vi "FPGA Target 2.vi"() -> ()   [LabVIEW 2025]
uses:
  <vilib>/Platform/TimedLoop/XDataNode/wakeup.ctl
  <vilib>/Platform/TimedLoop/XDataNode/XDNodeRunTimeDep.lvlib
  <vilib>/Platform/TimedLoop/XDataNode/nitl_modes.ctl
  <vilib>/Platform/TimedLoop/XDataNode/timing_clust.ctl
  <vilib>/Platform/TimedLoop/XDataNode/XDataNode.xnode
  SubModules/Engine Simulation Toolkit FPGA IP/IP Source/APU/APU.lvlib
  <vilib>/rvi/DataTransferAndStorage/Container/XNode/niFpgaContainer.xnode
  Templates/FPGA Wizard Templates.lvlib
  <vilib>/rvi/interface/RandomDataEmulation/nirviRandomDataFpgaReadWriteTemplate.vi
  SubModules/Engine Simulation Toolkit FPGA IP/IP Source/Digital Pattern Generation/Digital Pattern Generation.lvlib
  SubModules/Engine Simulation Toolkit FPGA IP/IP Source/Directional Speed/Directional Speed.lvlib
  SubModules/Engine Simulation Toolkit FPGA IP/IP Source/Analog Replay/Analog Replay.lvlib
  SubModules/FPGA Addon Speciality IO/Source/Speciality FPGA IO.lvlib
  SubModules/Engine Simulation Toolkit FPGA IP/IP Source/Knock Sensor/Knock Sensor.lvlib
  SubModules/Engine Simulation Toolkit FPGA IP/IP Source/ECU Event/Timing/ECU Event Timing.lvlib
  SubModules/Engine Simulation Toolkit FPGA IP/IP Source/ECU Event/Timing/Measure Events (Non-40MHz).vi
  SubModules/Engine Simulation Toolkit FPGA IP/IP Source/ECU Event/Timing/Capture Settings.ctl
  SubModules/Engine Simulation Toolkit FPGA IP/IP Source/APU/Shared Settings.ctl
  SubModules/Engine Simulation Toolkit FPGA IP/IP Source/Version Token.ctl
  SubModules/Engine Simulation Toolkit FPGA IP/IP Source/Engine Simulation Toolkit.lvlib
  SubModules/Engine Simulation Toolkit FPGA IP/IP Source/APU/Settings.ctl
  SubModules/Engine Simulation Toolkit FPGA IP/IP Source/APU/Input.ctl
  SubModules/Engine Simulation Toolkit FPGA IP/IP Source/APU/Output.ctl
  SubModules/Engine Simulation Toolkit FPGA IP/IP Source/Digital Pattern Generation/Load Input.ctl
  SubModules/Engine Simulation Toolkit FPGA IP/IP Source/Directional Speed/Load Input.ctl
  SubModules/Engine Simulation Toolkit FPGA IP/IP Source/Analog Replay/Load Input.ctl
  SubModules/FPGA Addon Speciality IO/Source/Types/PWM.Measure.Analog.Settings.ctl
  SubModules/FPGA Addon Speciality IO/Source/Types/PWM.Measure.Analog.Measurement.ctl
  SubModules/Engine Simulation Toolkit FPGA IP/IP Source/Knock Sensor/Cylinder Settings.ctl
  SubModules/Engine Simulation Toolkit FPGA IP/IP Source/Knock Sensor/Cylinder Input.ctl
  SubModules/Engine Simulation Toolkit FPGA IP/IP Source/Knock Sensor/Generate Settings.ctl
  SubModules/Engine Simulation Toolkit FPGA IP/IP Source/Knock Sensor/Generate Input.ctl
  SubModules/Engine Simulation Toolkit FPGA IP/IP Source/Analog Replay/Settings.ctl
  SubModules/Engine Simulation Toolkit FPGA IP/IP Source/Analog Replay/Input.ctl
  SubModules/FPGA Addon Speciality IO/Source/Types/Sine.Generate.Settings.ctl
  SubModules/FPGA Addon Speciality IO/Source/Types/PWM.Generate.Digital.Settings.ctl
  SubModules/Engine Simulation Toolkit FPGA IP/IP Source/Digital Pattern Generation/Settings.ctl
  SubModules/Engine Simulation Toolkit FPGA IP/IP Source/Digital Pattern Generation/Input.ctl
  SubModules/Engine Simulation Toolkit FPGA IP/IP Source/Directional Speed/Settings.ctl
  SubModules/Engine Simulation Toolkit FPGA IP/IP Source/Directional Speed/Input.ctl
  SubModules/FPGA Addon Speciality IO/Source/Types/WSS.Generate.Digital.Settings.ctl
  SubModules/FPGA Addon Speciality IO/Source/Types/Static.Generate.Digital.Settings.ctl
  SubModules/FPGA Addon Speciality IO/Source/Types/PWM.Measure.Digital.Settings.ctl
  SubModules/FPGA Addon Speciality IO/Source/Types/PWM.Measure.Digital.Measurement.ctl
  SubModules/Engine Simulation Toolkit FPGA IP/IP Source/ECU Event/Timing/Measure Settings.ctl
  SubModules/Engine Simulation Toolkit FPGA IP/IP Source/ECU Event/Timing/Measure Output.ctl
  SubModules/Engine Simulation Toolkit FPGA IP/IP Source/ECU Event/Timing/Capture Output.ctl
  SubModules/FPGA Addon Speciality IO/Source/Types/Static.Measure.Digital.Settings.ctl
  SubModules/FPGA Addon Speciality IO/Source/Types/Static.Measure.Digital.Measurement.ctl
panel:
  out "Ign Power Loopback.Measure":T1
  in  "Ign Power Loopback.Settings":T2={"ACTIVE EDGE"=TRUE}
  out "Accessory Loopback.Measure":T1
  in  "Accessory Loopback.Settings":T2={"ACTIVE EDGE"=TRUE}
  out "Front Driver WS Loopback.Measure":T1
  in  "Front Driver WS Loopback.Settings":T2={"ACTIVE EDGE"=TRUE}
  out "Mod4.Monitor":bool[](array[boolean])
  out "Crank Loopback.Measure":T1
  in  "Crank Loopback.Settings":T2={"ACTIVE EDGE"=TRUE}
  out "Crank_Temp Loopback.Measure":T1
  in  "Crank_Temp Loopback.Settings":T2={"ACTIVE EDGE"=TRUE}
  out "Switch Loopback":bool
  out "Key Loopback":bool
  out "capture.Exhaust CAM 1 Loopback.Event 4":T3
  out "capture.Exhaust CAM 1 Loopback.Event 3":T3
  out "capture.Exhaust CAM 1 Loopback.Event 2":T3
  out "capture.Exhaust CAM 1 Loopback.Event 1":T3
  out "status.Exhaust CAM 1 Loopback":T4
  in  "settings.Exhaust CAM 1 Loopback":T5
  out "capture.Intake CAM 1 Loopback.Event 4":T3
  out "capture.Intake CAM 1 Loopback.Event 3":T3
  out "capture.Intake CAM 1 Loopback.Event 2":T3
  out "capture.Intake CAM 1 Loopback.Event 1":T3
  out "status.Intake CAM 1 Loopback":T4
  in  "settings.Intake CAM 1 Loopback":T5
  out "PWM Out 2 Loopback.Measure":T6
  in  "PWM Out 2 Loopback.Settings":T7={"ACTIVE EDGE"=TRUE, "TIMEOUT"=40000000}
  out "PWM Out 1 Loopback.Measure":T6
  in  "PWM Out 1 Loopback.Settings":T7={"ACTIVE EDGE"=TRUE, "TIMEOUT"=40000000}
  out "Mod3.Monitor":bool[](array[boolean])
  out "Mod2.Monitor":bool[](array[boolean])
  in  "Ign Power.Settings":T8={"ACTIVE EDGE"=TRUE, "OUTPUT"=FALSE}
  in  "Accessory.Settings":T8={"ACTIVE EDGE"=TRUE, "OUTPUT"=FALSE}
  in  "Front Driver WS.Settings":T9={"ACTIVE EDGE"=TRUE, "ACTIVE TICKS"=0, "INACTIVE TICKS"=0, "DATA"=0, "SENSOR TYPE"=0}
  out "Mod1.Monitor":bool[](array[boolean])
  in  "input.Crank":T10
  in  "settings.Crank":T11
  in  "input.Crank_Temp":T12
  in  "settings.Crank_Temp":T13
  in  "Switch":bool
  in  "Key":bool
  in  "input.Exhaust CAM 1":T12
  in  "settings.Exhaust CAM 1":T13
  in  "input.Intake CAM 1":T12
  in  "settings.Intake CAM 1":T13
  in  "PWM Out 2.Settings":T14={"ACTIVE EDGE"=TRUE, "ACTIVE TICKS"=0, "INACTIVE TICKS"=0}
  in  "PWM Out 1.Settings":T14={"ACTIVE EDGE"=TRUE, "ACTIVE TICKS"=0, "INACTIVE TICKS"=0}
  out "Mod5.Monitor":fxp<+/-,32,8>[](array[numeric])
  in  "Simple Knock 2.Settings":T15={"AMP"=0.0, "OFFSET"=0.0, "PERIODS/TICKS"=2.4999957531690598e-05}
  in  "Simple Knock 1.Settings":T15={"AMP"=0.0, "OFFSET"=0.0, "PERIODS/TICKS"=2.4999957531690598e-05}
  in  "input.VR Sensor2":T16
  in  "settings.VR Sensor2":T17
  in  "input.VR Sensor1":T16
  in  "settings.VR Sensor1":T17
  in  "Power Supply Setpoint":fxp<+/-,32,8> format="%#_27g"
  in  "Dyno Setpoint":fxp<+/-,32,8> format="%#_27g"
  in  "input.Knock2":T18
  in  "settings.Knock2":T19
  in  "input.Knock2.Cylinder 6":T20={"probability compare"=65535, "high freq scaler"=0.0, "trigger position"=0}
  in  "settings.Knock2.Cylinder 6":T21
  in  "input.Knock2.Cylinder 5":T20={"probability compare"=65535, "high freq scaler"=0.0, "trigger position"=0}
  in  "settings.Knock2.Cylinder 5":T21
  in  "input.Knock2.Cylinder 4":T20={"probability compare"=65535, "high freq scaler"=0.0, "trigger position"=0}
  in  "settings.Knock2.Cylinder 4":T21
  in  "input.Knock2.Cylinder 3":T20={"probability compare"=65535, "high freq scaler"=0.0, "trigger position"=0}
  in  "settings.Knock2.Cylinder 3":T21
  in  "input.Knock2.Cylinder 2":T20={"probability compare"=65535, "high freq scaler"=0.0, "trigger position"=0}
  in  "settings.Knock2.Cylinder 2":T21
  in  "input.Knock2.Cylinder 1":T20={"probability compare"=65535, "high freq scaler"=0.0, "trigger position"=0}
  in  "settings.Knock2.Cylinder 1":T21
  in  "input.Knock1":T18
  in  "settings.Knock1":T19
  in  "input.Knock1.Cylinder 6":T20={"probability compare"=65535, "high freq scaler"=0.0, "trigger position"=0}
  in  "settings.Knock1.Cylinder 6":T21
  in  "input.Knock1.Cylinder 5":T20={"probability compare"=65535, "high freq scaler"=0.0, "trigger position"=0}
  in  "settings.Knock1.Cylinder 5":T21
  in  "input.Knock1.Cylinder 4":T20={"probability compare"=65535, "high freq scaler"=0.0, "trigger position"=0}
  in  "settings.Knock1.Cylinder 4":T21
  in  "input.Knock1.Cylinder 3":T20={"probability compare"=65535, "high freq scaler"=0.0, "trigger position"=0}
  in  "settings.Knock1.Cylinder 3":T21
  in  "input.Knock1.Cylinder 2":T20={"probability compare"=65535, "high freq scaler"=0.0, "trigger position"=0}
  in  "settings.Knock1.Cylinder 2":T21
  in  "input.Knock1.Cylinder 1":T20={"probability compare"=65535, "high freq scaler"=0.0, "trigger position"=0}
  in  "settings.Knock1.Cylinder 1":T21
  out "Simple Knock 2 Loopback":fxp<+/-,32,8> format="%#_27g"
  out "Simple Knock 1 Loopback":fxp<+/-,32,8> format="%#_27g"
  out "VR Sensor2 Loopback.Measure":T22
  in  "VR Sensor2 Loopback.Settings":T23={"ACTIVE EDGE"=TRUE, "TIMEOUT"=40000000, "THRESHOLD"=50.0}
  out "VR Sensor1 Loopback.Measure":T22
  in  "VR Sensor1 Loopback.Settings":T23={"ACTIVE EDGE"=TRUE, "TIMEOUT"=40000000, "THRESHOLD"=50.0}
  out "Power Supply Setpoint Loopback":fxp<+/-,32,8> format="%#_27g"
  out "Dyno Setpoint Loopback":fxp<+/-,32,8> format="%#_27g"
  out "Knock2 Loopback":fxp<+/-,32,8> format="%#_27g"
  out "Knock1 Loopback":fxp<+/-,32,8> format="%#_27g"
  out "Mod6.Monitor":fxp<+/-,24,5>[](array[numeric])
  in  "load input.VR Sensor2":T24={"Data"=[0, 0, 0, 0, 0, 0, 0, 0, 0, 0, 0, 0, 0, 0, 0, 0], "LoadOffset"=0, "Done"=FALSE}
  in  "load input.VR Sensor1":T24={"Data"=[0, 0, 0, 0, 0, 0, 0, 0, 0, 0, 0, 0, 0, 0, 0, 0], "LoadOffset"=0, "Done"=FALSE}
  in  "load input.Crank":T25
  in  "load input.Crank_Temp":T26
  in  "load input.Exhaust CAM 1":T26
  in  "load input.Intake CAM 1":T26
  out "Actual Analog Input Loop Period (usec)":u32
  out "Actual Analog Output Loop Period (usec)":u32
  out "Actual Digital Loop Period (usec)":u32
  out "Actual DMA Loop Period (usec)":u32
  in  "Analog Input Loop Timer (uSec)":u32=10
  out "output.apu 1":T27 caption="output"
  in  "input.apu 1":T28={"desired speed"=0.0, "reset"=TRUE} caption="input"
  in  "settings.apu 1":T29 caption="settings"
  in  "est.version":T30
  in  "shared settings.apu 1":T31 {"start" format="%#.15g"}
  in  "go.apu 1":bool
  in  "Digital Loop Timer (uSec)":u32=10
  in  "Analog Output Loop Timer (uSec)":u32=10
  in  "DMA.Enable":bool
  in  "DMA.MinimumSamples":u32=100000 caption="DMA Loop Timer (uSec)"
  out "DMA.Timeout":bool
  in  "DMA.Timeout.Reset":bool
  in  "DMA Loop Timer (uSec)":u32=10
types:
  T1 = typedef "Speciality FPGA IO.lvlib/Static.Measure.Digital.Measurement.ctl" = cluster{"STATE":bool}
  T2 = typedef "Speciality FPGA IO.lvlib/Static.Measure.Digital.Settings.ctl" = cluster{"ACTIVE EDGE":bool}
  T3 = typedef "Engine Simulation Toolkit.lvlib/ECU Event Timing.lvlib/Capture Output.ctl" = cluster{"Start":u16, "End":u16, "Duration (tics)":fxp<+,18,18>, "Event present":bool}
  T4 = typedef "Engine Simulation Toolkit.lvlib/ECU Event Timing.lvlib/Measure Output.ctl" = cluster{"stuck active":bool, "window all active":bool, "window orphan start":bool, "window orphan end":bool}
  T5 = typedef "Engine Simulation Toolkit.lvlib/ECU Event Timing.lvlib/Measure Settings.ctl" = cluster{"max":u16, "min":u16, "active high":bool, "wrap":bool}
  T6 = typedef "Speciality FPGA IO.lvlib/PWM.Measure.Digital.Measurement.ctl" = cluster{"ACTIVE TICKS":u32, "INACTIVE TICKS":u32, "ACQ TICKS":u32}
  T7 = typedef "Speciality FPGA IO.lvlib/PWM.Measure.Digital.Settings.ctl" = cluster{"ACTIVE EDGE":bool, "TIMEOUT":u32}
  T8 = typedef "Speciality FPGA IO.lvlib/Static.Generate.Digital.Settings.ctl" = cluster{"ACTIVE EDGE":bool, "OUTPUT":bool}
  T9 = typedef "Speciality FPGA IO.lvlib/WSS.Generate.Digital.Settings.ctl" = cluster{"ACTIVE EDGE":bool, "ACTIVE TICKS":u32, "INACTIVE TICKS":u32, "DATA":u8, "SENSOR TYPE":u8}
  T10 = typedef "Engine Simulation Toolkit.lvlib/Directional Speed.lvlib/Input.ctl" = cluster{"td (tics)":u16, "tf (tics)":u16, "tr (tics)":u16}
  T11 = typedef "Engine Simulation Toolkit.lvlib/Directional Speed.lvlib/Settings.ctl" = cluster{"Upper Value":u16, "Lower Value":u16, "Upper Index":fxp<+,10,10>, "Lower Index":fxp<+,10,10>, "Enabled":bool}
  T12 = typedef "Engine Simulation Toolkit.lvlib/Digital Pattern Generation.lvlib/Input.ctl" = cluster{"Offset":i16}
  T13 = typedef "Engine Simulation Toolkit.lvlib/Digital Pattern Generation.lvlib/Settings.ctl" = cluster{"edge 1":u16, "edge 2":u16, "cycle angle":bool, "enabled":bool, "first falling":bool, "fault":bool, "fault wrap":bool, "fault value":bool, "fault count":fxp<+,4,4>, "use fault count":bool}
  T14 = typedef "Speciality FPGA IO.lvlib/PWM.Generate.Digital.Settings.ctl" = cluster{"ACTIVE EDGE":bool, "ACTIVE TICKS":u32, "INACTIVE TICKS":u32}
  T15 = typedef "Speciality FPGA IO.lvlib/Sine.Generate.Settings.ctl" = cluster{"AMP":fxp<+/-,32,8>, "OFFSET":fxp<+/-,32,8>, "PERIODS/TICKS":fxp<+,32,0>}
  T16 = typedef "Engine Simulation Toolkit.lvlib/Analog Replay.lvlib/Input.ctl" = cluster{"Offset":i16, "VScaleSlope":fxp<+,18,6>, "VScaleIntercept":fxp<+/-,18,3>}
  T17 = typedef "Engine Simulation Toolkit.lvlib/Analog Replay.lvlib/Settings.ctl" = cluster{"ReverseNegate":bool, "CycleAngle":bool, "SpeedThreshold":fxp<+/-,23,2>, "AOBelowThreshold":i16}
  T18 = typedef "Engine Simulation Toolkit.lvlib/Knock Sensor.lvlib/Generate Input.ctl" = cluster{"low freq scaler":fxp<+,10,0>}
  T19 = typedef "Engine Simulation Toolkit.lvlib/Knock Sensor.lvlib/Generate Settings.ctl" = cluster{"low freq (periods/tick)":fxp<+,32,0>, "high freq (periods/tick)":fxp<+,32,0>, "duration (1.25MHz tics)":fxp<+,18,18>, "low freq speed slope":fxp<+,16,-3>, "low freq speed intercept":fxp<+,10,-10>, "low freq by speed":bool}
  T20 = typedef "Engine Simulation Toolkit.lvlib/Knock Sensor.lvlib/Cylinder Input.ctl" = cluster{"probability compare":u16, "high freq scaler":fxp<+,10,0>, "trigger position":u16}
  T21 = typedef "Engine Simulation Toolkit.lvlib/Knock Sensor.lvlib/Cylinder Settings.ctl" = cluster{"seed":u16, "reset":bool}
  T22 = typedef "Speciality FPGA IO.lvlib/PWM.Measure.Analog.Measurement.ctl" = cluster{"ACTIVE TICKS":u32, "INACTIVE TICKS":u32, "ACQ TICKS":u32, "ACTIVE VOLTAGE":fxp<+/-,32,8>, "INACTIVE VOLTAGE":fxp<+/-,32,8>}
  T23 = typedef "Speciality FPGA IO.lvlib/PWM.Measure.Analog.Settings.ctl" = cluster{"ACTIVE EDGE":bool, "TIMEOUT":u32, "THRESHOLD":fxp<+/-,32,8>}
  T24 = typedef "Engine Simulation Toolkit.lvlib/Analog Replay.lvlib/Load Input.ctl" = cluster{"Data":i16[], "LoadOffset":u16, "Done":bool}
  T25 = typedef "Engine Simulation Toolkit.lvlib/Directional Speed.lvlib/Load Input.ctl" = cluster{"address":fxp<+,10,10>, "done":bool, "angle":u16}
  T26 = typedef "Engine Simulation Toolkit.lvlib/Digital Pattern Generation.lvlib/Load Input.ctl" = cluster{"address":fxp<+,11,11>, "done":bool, "angle":u16}
  T27 = typedef "Engine Simulation Toolkit.lvlib/APU.lvlib/Output.ctl" = cluster{"crank":u16, "cycle":u16, "actual speed":fxp<+/-,23,2>}
  T28 = typedef "Engine Simulation Toolkit.lvlib/APU.lvlib/Input.ctl" = cluster{"desired speed":fxp<+/-,23,2>, "reset":bool}
  T29 = typedef "Engine Simulation Toolkit.lvlib/APU.lvlib/Settings.ctl" = cluster{"acceleration":fxp<+,18,-20>, "enable accel":bool}
  T30 = typedef "Engine Simulation Toolkit.lvlib/Version Token.ctl" = cluster{"1.4.0":bool}
  T31 = typedef "Engine Simulation Toolkit.lvlib/APU.lvlib/Shared Settings.ctl" = cluster{"start":fxp<+,17,17>, "stuck limit":fxp<+,18,18>}
  T32 = typedef "XDNodeRunTimeDep.lvlib/timing_clust.ctl" = cluster{"Expected End [f-1]":u64, "Actual End [f-1]":u64, "Finished Late? [f-1]":bool, "Expected End [i-1]":u64, "Actual End [i-1]":u64, "Finished Late? [i-1]":bool, "Expected Start [i]":u64, "Actual Start [i]":u64, "Expected Start [f]":u64, "Actual Start [f]":u64, "Source Name":string, "Structure Name":string, "Period":i64, "Deadline":i64, "Offset":i64, "Start":i64, "Priority":i32, "Timeout":i32, "Mode":T33, "Wakeup Reason":T34, "Error":errorcluster, "Source Type":string, "Secondary Source Type":string, "Global End Time":u64, "Global Start Time":u64, "Frame Duration":u64, "Iteration Duration":u64, "Assigned CPU":i32, "I/O Scan Engine Mode":u32}
  T33 = typedef "XDNodeRunTimeDep.lvlib/nitl_modes.ctl" = enum32{"No Change", "Process missed periods, maintain original phase", "Discard missed periods, maintain original phase", "Process missed periods, ignore original phase", "Discard missed periods, ignore original phase"}
  T34 = typedef "XDNodeRunTimeDep.lvlib/wakeup.ctl" = enum32{"Normal", "Aborted", "Asynchronous wakeup", "Timing source error", "Timed loop error", "Timeout"}
  T35 = cluster{"DI 0":refnum<k21>, "DI 1":refnum<k21>, "DI 2":refnum<k21>, "DI 3":refnum<k21>, "DI 4":refnum<k21>, "DI 5":refnum<k21>, "DI 6":refnum<k21>, "DI 7":refnum<k21>}
  T36 = typedef "Engine Simulation Toolkit.lvlib/ECU Event Timing.lvlib/Capture Settings.ctl" = u8
  T37 = cluster{"DO 0":refnum<k21>, "DO 1":refnum<k21>, "DO 2":refnum<k21>, "DO 3":refnum<k21>, "DO 4":refnum<k21>, "DO 5":refnum<k21>, "DO 6":refnum<k21>, "DO 7":refnum<k21>}
  T38 = cluster{"AO 0":refnum<k21>, "AO 1":refnum<k21>, "AO 2":refnum<k21>, "AO 3":refnum<k21>, "AO 4":refnum<k21>, "AO 5":refnum<k21>, "AO 6":refnum<k21>, "AO 7":refnum<k21>, "AO 8":refnum<k21>, "AO 9":refnum<k21>, "AO 10":refnum<k21>, "AO 11":refnum<k21>, "AO 12":refnum<k21>, "AO 13":refnum<k21>, "AO 14":refnum<k21>, "AO 15":refnum<k21>}
  T39 = cluster{"AI 0":refnum<k21>, "AI 1":refnum<k21>, "AI 2":refnum<k21>, "AI 3":refnum<k21>, "AI 4":refnum<k21>, "AI 5":refnum<k21>, "AI 6":refnum<k21>, "AI 7":refnum<k21>, "AI 8":refnum<k21>, "AI 9":refnum<k21>, "AI 10":refnum<k21>, "AI 11":refnum<k21>, "AI 12":refnum<k21>, "AI 13":refnum<k21>, "AI 14":refnum<k21>, "AI 15":refnum<k21>}
  T40 = typedef "Engine Simulation Toolkit.lvlib/Digital Pattern Generation.lvlib/Load Data.ctl" = cluster{"max address":fxp<+,11,11>, "memory":refnum<k21>}
  T41 = typedef "Engine Simulation Toolkit.lvlib/Directional Speed.lvlib/Load Data.ctl" = cluster{"max address":fxp<+,10,10>, "Memory":refnum<k21>}
  T42 = typedef "Engine Simulation Toolkit.lvlib/APU.lvlib/Register Bus.ctl" = cluster{"Speed":refnum<k21>, "Crank Angle":refnum<k21>, "Cycle Angle":refnum<k21>, "Crank Count":refnum<k21>, "Cycle Count":refnum<k21>, "1.25 MHz Counter":refnum<k21>, "Crank Rollover":refnum<k21>, "Cycle Rollover":refnum<k21>, "shared settings":T31}
  T43 = typedef "Engine Simulation Toolkit.lvlib/Knock Sensor.lvlib/Triggered Cylinder Data.ctl" = cluster{"trigger knock":bool, "high freq scaler":fxp<+,10,0>}
  T44 = typedef "Engine Simulation Toolkit.lvlib/ECU Event Timing.lvlib/Measured Data.ctl" = cluster{"start":u16, "end":u16, "duration (tics)":fxp<+,18,18>, "window end":bool, "window begin":bool, "pulse end":bool, "pulse #":u8}
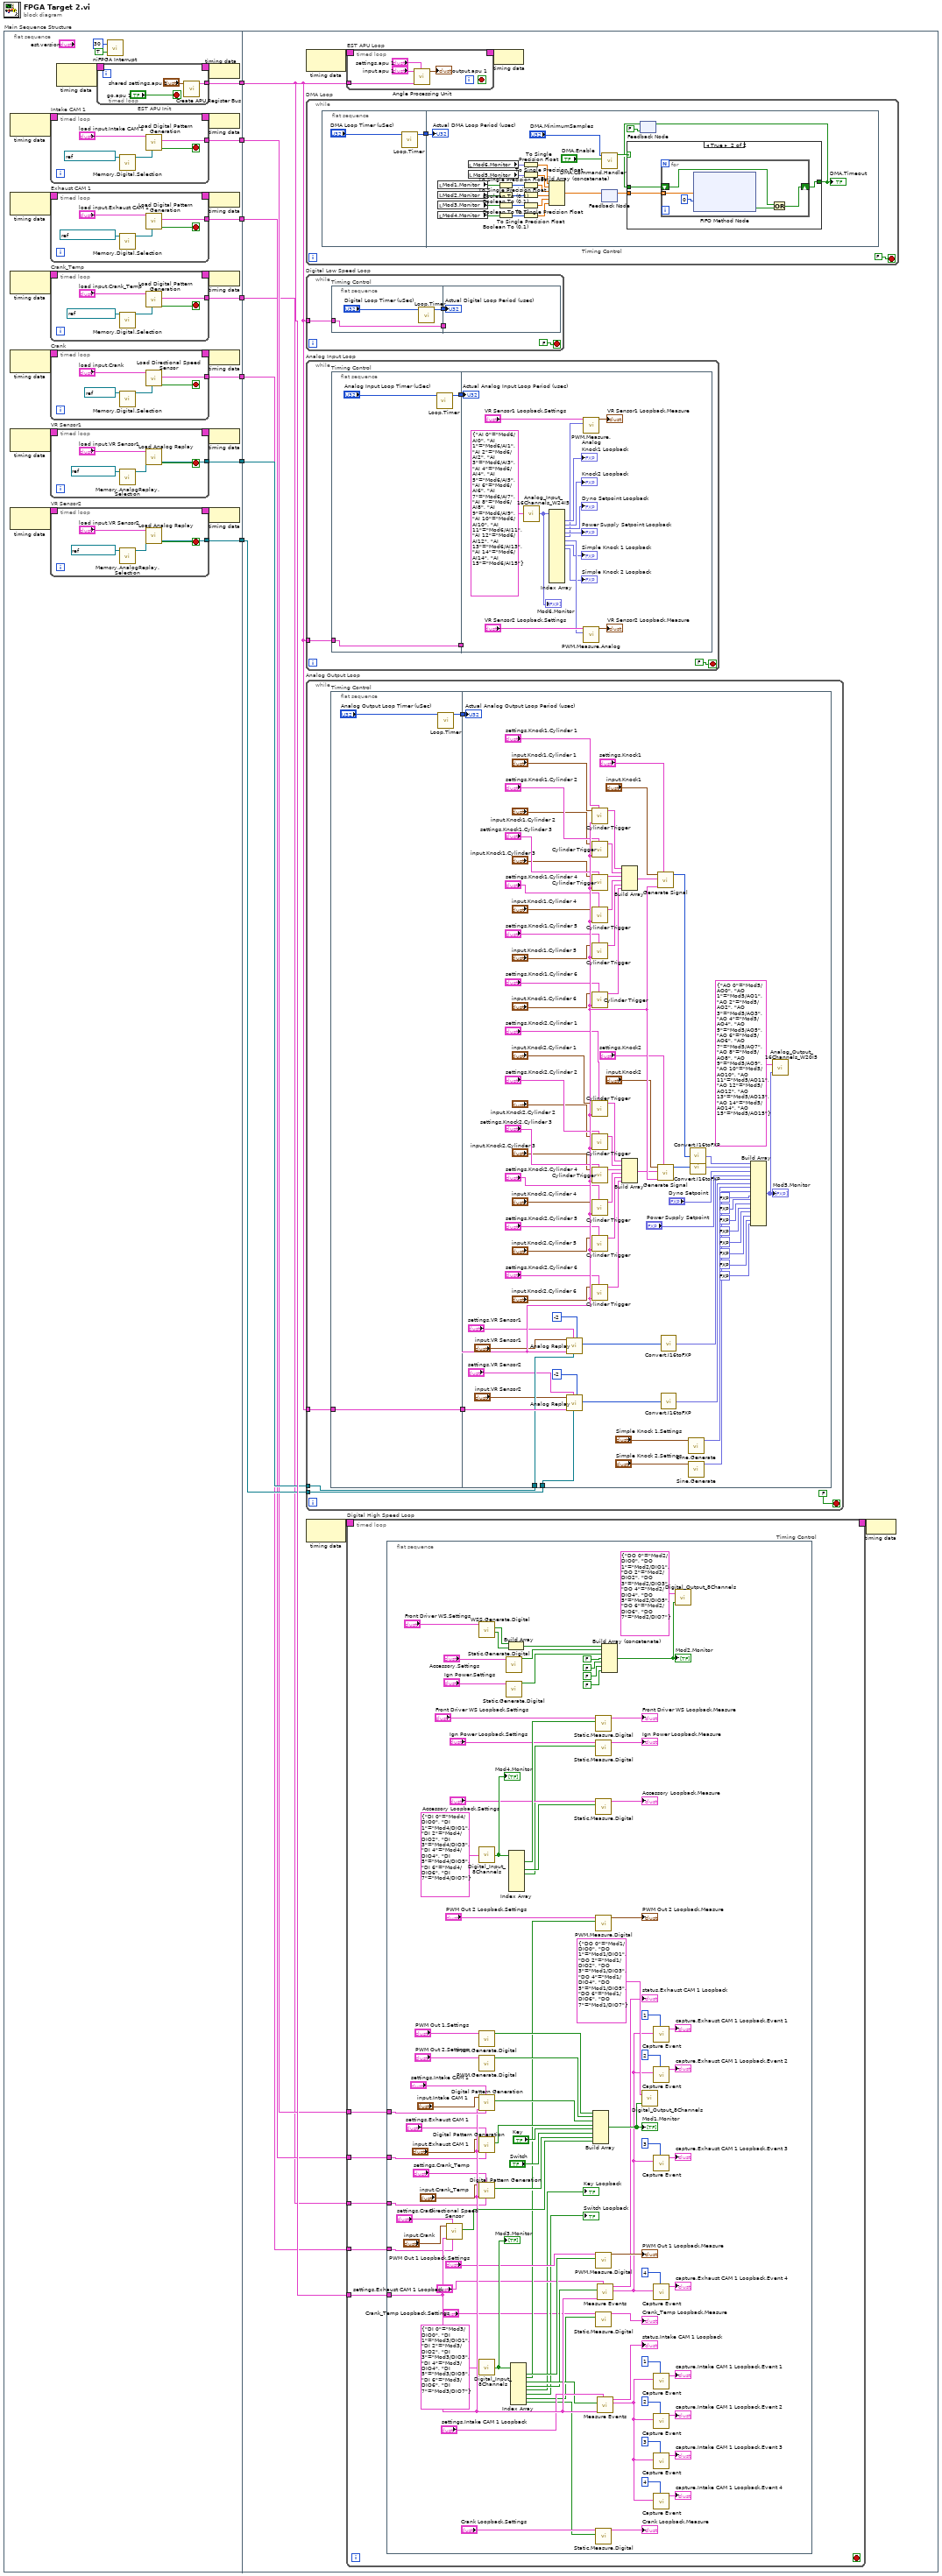
[diagram p0: block diagram]
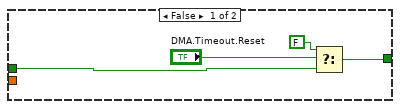
[diagram p2: hidden frame]
diagram:
  n1 = flat-sequence "Main Sequence Structure" {
    tunnel: [w26] -> w7
    tunnel: [w13] -> w6
    tunnel: [w12] -> w5
    tunnel: [w11] -> w4
    tunnel: [w10] -> w3
    tunnel: [w9] -> w2
    tunnel: [w8] -> w1
    tunnel: w7 -> [w96]
    tunnel: w6 -> [w95]
    tunnel: w5 -> [w94]
    tunnel: w4 -> [w93]
    tunnel: w3 -> [w92]
    tunnel: w2 -> [w91]
    tunnel: w1 -> [w90]
    frame #0 {
      n2 = node-c288() -> (w25:T32)  [unwired: 1 in]
      n3 = node-c288() -> (w23:T32)  [unwired: 1 in]
      n4 = node-c288() -> (w21:T32)  [unwired: 1 in]
      n5 = node-c288() -> (w19:T32)  [unwired: 1 in]
      n6 = node-c288() -> (w17:T32)  [unwired: 1 in]
      n7 = node-c288() -> (w15:T32)  [unwired: 1 in]
      n8 = timed-loop "Intake CAM 1" {
        timing: w25 -> [_]
        timing-out: [_] -> w24
        tunnel: [w74] -> w11
        stop <- w77 stop-if-true
        n9 = call "Memory.Digital.Selection.vi"("memory"=refnum<k21> "Intake CAM 1") -> ("memory"=w75:refnum<k21>)  [unwired: 10 in]
        n10 = call "Load Digital Pattern Generation.vi"("memory"=w75, "load input.<user name>"="load input.Intake CAM 1") -> ("done"=w77:bool, "load data"=w74:T40)  [unwired: 8 in]
      }
      n11 = timed-loop "Exhaust CAM 1" {
        timing: w23 -> [_]
        timing-out: [_] -> w22
        tunnel: [w65] -> w10
        stop <- w68 stop-if-true
        n12 = call "Memory.Digital.Selection.vi"("memory"=refnum<k21> "Exhaust CAM 1") -> ("memory"=w66:refnum<k21>)  [unwired: 10 in]
        n13 = call "Load Digital Pattern Generation.vi"("memory"=w66, "load input.<user name>"="load input.Exhaust CAM 1") -> ("done"=w68:bool, "load data"=w65:T40)  [unwired: 8 in]
      }
      n14 = timed-loop "Crank_Temp" {
        timing: w21 -> [_]
        timing-out: [_] -> w20
        tunnel: [w56] -> w9
        stop <- w59 stop-if-true
        n15 = call "Memory.Digital.Selection.vi"("memory"=refnum<k21> "Crank_Temp") -> ("memory"=w57:refnum<k21>)  [unwired: 10 in]
        n16 = call "Load Digital Pattern Generation.vi"("memory"=w57, "load input.<user name>"="load input.Crank_Temp") -> ("done"=w59:bool, "load data"=w56:T40)  [unwired: 8 in]
      }
      n17 = timed-loop "Crank" {
        timing: w19 -> [_]
        timing-out: [_] -> w18
        tunnel: [w47] -> w8
        stop <- w50 stop-if-true
        n18 = call "Memory.Digital.Selection.vi"("memory"=refnum<k21> "Crank") -> ("memory"=w48:refnum<k21>)  [unwired: 10 in]
        n19 = call "Load Directional Speed Sensor.vi"("Memory In"=w48, "load input.<user name>"="load input.Crank") -> ("done"=w50:bool, "load data"=w47:T41)  [unwired: 8 in]
      }
      n20 = timed-loop "VR Sensor1" {
        timing: w17 -> [_]
        timing-out: [_] -> w16
        tunnel: [w39] -> w13
        stop <- w41 stop-if-true
        n21 = call "Memory.AnalogReplay.Selection.vi"("memory"=refnum<k21> "VR Sensor1") -> ("memory"=w39:refnum<k21>)  [unwired: 10 in]
        n22 = call "Load Analog Replay.vi"("memory"=w39, "load input.<user name>"="load input.VR Sensor1") -> ("done"=w41:bool)  [unwired: 9 in]
      }
      n23 = timed-loop "VR Sensor2" {
        timing: w15 -> [_]
        timing-out: [_] -> w14
        tunnel: [w31] -> w12
        stop <- w33 stop-if-true
        n24 = call "Memory.AnalogReplay.Selection.vi"("memory"=refnum<k21> "VR Sensor2") -> ("memory"=w31:refnum<k21>)  [unwired: 10 in]
        n25 = call "Load Analog Replay.vi"("memory"=w31, "load input.<user name>"="load input.VR Sensor2") -> ("done"=w33:bool)  [unwired: 9 in]
      }
      n26 = node-c288() -> (w28:T32)  [unwired: 1 in]
      n27 = timed-loop "EST APU Init" {
        timing: w28 -> [_]
        timing-out: [_] -> w27
        tunnel: [w83] -> w26
        stop <- "go.apu 1" stop-if-true
        n28 = call "Create APU Register Bus.vi"("shared settings.<user name>"="shared settings.apu 1") -> ("register bus"=w83:T42)  [unwired: 10 in]
      }
      n29 = call <vilib>:"niFPGA Interrupt.vi"("Wait Until Cleared (F)"=TRUE, "IRQ Number (0)"=u8 30) -> ()  [unwired: 1 in]
      n30 = node-c288(w27) -> ()
      n31 = node-c288(w24) -> ()
      n32 = node-c288(w22) -> ()
      n33 = node-c288(w20) -> ()
      n34 = node-c288(w18) -> ()
      n35 = node-c288(w16) -> ()
      n36 = node-c288(w14) -> ()
    }
    frame #1 {
      # "FPGA Addon Code"
      n37 = node-c288 ("Input Node")() -> (w98:T32)  [unwired: 1 in]
      n38 = while "DMA Loop" {
        stop <- FALSE stop-if-true
        n39 = flat-sequence "Timing Control" {
          tunnel: [w210] -> w208
          tunnel: w208 -> [w228]
          frame #0 {
            n40 = call "Loop.Timer.vi"("Loop Timer (uSec)"="DMA Loop Timer (uSec)") -> ("Actual Loop Period (usec)"=w210:u32)  [unwired: 10 in]
          }
          frame #1 {
            n41 = local read "Mod1.Monitor"() -> (w225:bool[])
            n42 = local read "Mod2.Monitor"() -> (w223:bool[])
            n43 = local read "Mod3.Monitor"() -> (w221:bool[])
            n44 = local read "Mod4.Monitor"() -> (w219:bool[])
            n45 = local read "Mod6.Monitor"() -> (w227:fxp<+/-,24,5>[])
            n46 = local read "Mod5.Monitor"() -> (w226:fxp<+/-,32,8>[])
            n47 = Boolean To (0,1)(Boolean=w225) -> (0, 1=w224:i16[])
            n48 = Boolean To (0,1)(Boolean=w223) -> (0, 1=w222:i16[])
            n49 = Boolean To (0,1)(Boolean=w221) -> (0, 1=w220:i16[])
            n50 = Boolean To (0,1)(Boolean=w219) -> (0, 1=w218:i16[])
            n51 = To Single Precision Float(number=w227) -> (single precision float=w217:sgl[])
            n52 = To Single Precision Float(number=w226) -> (single precision float=w216:sgl[])
            n53 = To Single Precision Float(number=w224) -> (single precision float=w215:sgl[])
            n54 = To Single Precision Float(number=w222) -> (single precision float=w214:sgl[])
            n55 = To Single Precision Float(number=w220) -> (single precision float=w213:sgl[])
            n56 = To Single Precision Float(number=w218) -> (single precision float=w212:sgl[])
            n57 = Build Array (concatenate) "Build Array"(w217, w216, w215, w214, w213, w212) -> (w234:sgl[])
            n58 = call "DMA.Command.Handler.vi"("DMA.Enable"="DMA.Enable", "DMA.MinimumSamples"="DMA.MinimumSamples") -> ("Transfer"=w230:bool)  [unwired: 9 in]
            n59 = feedback #1() -> (w233:sgl[])  [unwired: 1 in]
            n60 = feedback-in #1(w234) -> ()
            n61 = feedback #2(FALSE ("t")) -> (w229:bool)
            n62 = case shown="True" w230 {
              tunnel: w233 -> [_ w243]
              tunnel: w229 -> [w238 w242]
              tunnel: [w237 w241] -> w232
              frame False {
                n63 = Select(t=FALSE, s="DMA.Timeout.Reset", f=w238) -> (s? t:f=w237:bool)
              }
              frame True {
                n64 = for {
                  shift-right: [w246] -> w241
                  shift-left: w242 -> [w245]
                  tunnel: w243 -> [w244] mode=indexing
                  n65 = xnode ("FIFO Method Node")("Element"=w244, "Timeout"=0) -> ("Timed Out?"=w247:bool)  [unwired: 1 in, 1 out]
                  n66 = Or(x=w245, y=w247) -> (x .or. y?=w246:bool)
                }
              }
            }
            "DMA.Timeout" <- w232
            n67 = feedback-in #2(w232) -> ()
            "Actual DMA Loop Period (usec)" <- w228
          }
        }
      }
      n68 = while "Digital Low Speed Loop" {
        tunnel: w96 -> [w358]
        stop <- FALSE stop-if-true
        n69 = flat-sequence "Timing Control" {
          tunnel: w358 -> [w362]
          tunnel: [w362] -> w357
          tunnel: [w360] -> w356
          tunnel: w357 -> [_]
          tunnel: w356 -> [w363]
          frame #0 {
            n70 = call "Loop.Timer.vi"("Loop Timer (uSec)"="Digital Loop Timer (uSec)") -> ("Actual Loop Period (usec)"=w360:u32)  [unwired: 10 in]
          }
          frame #1 {
            "Actual Digital Loop Period (usec)" <- w363
          }
        }
      }
      n71 = while "Analog Input Loop" {
        tunnel: w96 -> [w336]
        stop <- FALSE stop-if-true
        n72 = flat-sequence "Timing Control" {
          tunnel: w336 -> [w340]
          tunnel: [w340] -> w335
          tunnel: [w338] -> w334
          tunnel: w335 -> [_]
          tunnel: w334 -> [w355]
          frame #0 {
            n73 = call "Loop.Timer.vi"("Loop Timer (uSec)"="Analog Input Loop Timer (uSec)") -> ("Actual Loop Period (usec)"=w338:u32)  [unwired: 10 in]
          }
          frame #1 {
            n74 = call "Analog_Input_16Channels_W24I5.vi"("IO"=T39 {"AI 0"="Mod6/AI0", "AI 1"="Mod6/AI1", "AI 2"="Mod6/AI2", "AI 3"="Mod6/AI3", "AI 4"="Mod6/AI4", "AI 5"="Mod6/AI5", "AI 6"="Mod6/AI6", "AI 7"="Mod6/AI7", "AI 8"="Mod6/AI8", "AI 9"="Mod6/AI9", "AI 10"="Mod6/AI10", "AI 11"="Mod6/AI11", "AI 12"="Mod6/AI12", "AI 13"="Mod6/AI13", "AI 14"="Mod6/AI14", "AI 15"="Mod6/AI15"}) -> ("Values"=w353:fxp<+/-,24,5>[])
            "Mod6.Monitor" <- w353
            n75 = Index Array(array=w353) -> (element #1=→"Knock1 Loopback":fxp<+/-,24,5>, element #2=→"Knock2 Loopback":fxp<+/-,24,5>, element #3=→"Dyno Setpoint Loopback":fxp<+/-,24,5>, element #4=→"Power Supply Setpoint Loopback":fxp<+/-,24,5>, element #5=w347:fxp<+/-,24,5>, element #6=w344:fxp<+/-,24,5>, element #7=→"Simple Knock 1 Loopback":fxp<+/-,24,5>, element #8=→"Simple Knock 2 Loopback":fxp<+/-,24,5>)  [unwired: 16 in, 8 out]
            n76 = call "PWM.Measure.Analog.vi"("PWM"=w347, "Settings"="VR Sensor1 Loopback.Settings") -> ("Measurement"=→"VR Sensor1 Loopback.Measure":T22)  [unwired: 8 in, 1 out]
            n77 = call "PWM.Measure.Analog.vi"("PWM"=w344, "Settings"="VR Sensor2 Loopback.Settings") -> ("Measurement"=→"VR Sensor2 Loopback.Measure":T22)  [unwired: 8 in, 1 out]
            "Actual Analog Input Loop Period (usec)" <- w355
          }
        }
      }
      n78 = while "Analog Output Loop" {
        tunnel: w96 -> [w253]
        tunnel: w95 -> [w250]
        tunnel: w94 -> [w249]
        stop <- FALSE stop-if-true
        n79 = flat-sequence "Timing Control" {
          tunnel: w253 -> [w257]
          tunnel: [w257] -> w252
          tunnel: [w255] -> w251
          tunnel: w252 -> [w330]
          tunnel: w251 -> [w333]
          tunnel: w250 -> [w284]
          tunnel: w249 -> [w279]
          frame #0 {
            n80 = call "Loop.Timer.vi"("Loop Timer (uSec)"="Analog Output Loop Timer (uSec)") -> ("Actual Loop Period (usec)"=w255:u32)  [unwired: 10 in]
          }
          frame #1 {
            n81 = call "Analog Replay.vi"("shift"=i8 -2, "memory"=w284, "settings.<user name>"="settings.VR Sensor1", "register bus"=w330, "input.<user name>"="input.VR Sensor1") -> ("analog value"=w283:i16)  [unwired: 6 in]
            n82 = call "Analog Replay.vi"("shift"=i8 -2, "memory"=w279, "settings.<user name>"="settings.VR Sensor2", "register bus"=w330, "input.<user name>"="input.VR Sensor2") -> ("analog value"=w278:i16)  [unwired: 6 in]
            n83 = call "Cylinder Trigger.vi"("settings.<user name>"="settings.Knock1.Cylinder 1", "register bus"=w330, "input.<user name>"="input.Knock1.Cylinder 1") -> ("triggered knock data"=w329:T43)  [unwired: 8 in]
            n84 = call "Cylinder Trigger.vi"("settings.<user name>"="settings.Knock1.Cylinder 2", "register bus"=w330, "input.<user name>"="input.Knock1.Cylinder 2") -> ("triggered knock data"=w326:T43)  [unwired: 8 in]
            n85 = call "Cylinder Trigger.vi"("settings.<user name>"="settings.Knock1.Cylinder 3", "register bus"=w330, "input.<user name>"="input.Knock1.Cylinder 3") -> ("triggered knock data"=w323:T43)  [unwired: 8 in]
            n86 = call "Cylinder Trigger.vi"("settings.<user name>"="settings.Knock1.Cylinder 4", "register bus"=w330, "input.<user name>"="input.Knock1.Cylinder 4") -> ("triggered knock data"=w320:T43)  [unwired: 8 in]
            n87 = call "Cylinder Trigger.vi"("settings.<user name>"="settings.Knock1.Cylinder 5", "register bus"=w330, "input.<user name>"="input.Knock1.Cylinder 5") -> ("triggered knock data"=w317:T43)  [unwired: 8 in]
            n88 = call "Cylinder Trigger.vi"("settings.<user name>"="settings.Knock1.Cylinder 6", "register bus"=w330, "input.<user name>"="input.Knock1.Cylinder 6") -> ("triggered knock data"=w314:T43)  [unwired: 8 in]
            n89 = call "Cylinder Trigger.vi"("settings.<user name>"="settings.Knock2.Cylinder 1", "register bus"=w330, "input.<user name>"="input.Knock2.Cylinder 1") -> ("triggered knock data"=w307:T43)  [unwired: 8 in]
            n90 = call "Cylinder Trigger.vi"("settings.<user name>"="settings.Knock2.Cylinder 2", "register bus"=w330, "input.<user name>"="input.Knock2.Cylinder 2") -> ("triggered knock data"=w304:T43)  [unwired: 8 in]
            n91 = call "Cylinder Trigger.vi"("settings.<user name>"="settings.Knock2.Cylinder 3", "register bus"=w330, "input.<user name>"="input.Knock2.Cylinder 3") -> ("triggered knock data"=w301:T43)  [unwired: 8 in]
            n92 = call "Cylinder Trigger.vi"("settings.<user name>"="settings.Knock2.Cylinder 4", "register bus"=w330, "input.<user name>"="input.Knock2.Cylinder 4") -> ("triggered knock data"=w298:T43)  [unwired: 8 in]
            n93 = call "Cylinder Trigger.vi"("settings.<user name>"="settings.Knock2.Cylinder 5", "register bus"=w330, "input.<user name>"="input.Knock2.Cylinder 5") -> ("triggered knock data"=w295:T43)  [unwired: 8 in]
            n94 = call "Cylinder Trigger.vi"("settings.<user name>"="settings.Knock2.Cylinder 6", "register bus"=w330, "input.<user name>"="input.Knock2.Cylinder 6") -> ("triggered knock data"=w292:T43)  [unwired: 8 in]
            n95 = Build Array(w329, w326, w323, w320, w317, w314) -> (w311:T43[])
            n96 = Build Array(w307, w304, w301, w298, w295, w292) -> (w289:T43[])
            n97 = call "Generate Signal.vi"("settings.<user name>"="settings.Knock1", "register bus"=w330, "triggered knock data"=w311, "input.<user name>"="input.Knock1") -> ("knock signal"=w310:i16)  [unwired: 7 in]
            n98 = call "Generate Signal.vi"("settings.<user name>"="settings.Knock2", "register bus"=w330, "triggered knock data"=w289, "input.<user name>"="input.Knock2") -> ("knock signal"=w288:i16)  [unwired: 7 in]
            n99 = call "Convert.I16toFXP.vi"("16bit integer"=w283) -> ("x*y"=w271:fxp<+/-,20,5>)  [unwired: 4 in]
            n100 = call "Convert.I16toFXP.vi"("16bit integer"=w278) -> ("x*y"=w270:fxp<+/-,20,5>)  [unwired: 4 in]
            n101 = call "Sine.Generate.vi"("Settings"="Simple Knock 1.Settings") -> ("Output"=w269:fxp<+/-,32,8>)  [unwired: 10 in]
            n102 = call "Sine.Generate.vi"("Settings"="Simple Knock 2.Settings") -> ("Output"=w268:fxp<+/-,32,8>)  [unwired: 10 in]
            n103 = call "Convert.I16toFXP.vi"("16bit integer"=w310) -> ("x*y"=w275:fxp<+/-,20,5>)  [unwired: 4 in]
            n104 = call "Convert.I16toFXP.vi"("16bit integer"=w288) -> ("x*y"=w274:fxp<+/-,20,5>)  [unwired: 4 in]
            n105 = Build Array(w275, w274, "Dyno Setpoint", "Power Supply Setpoint", w271, w270, w269, w268, fxp<+/-,32,8> 0.0, fxp<+/-,32,8> 0.0, fxp<+/-,32,8> 0.0, fxp<+/-,32,8> 0.0, fxp<+/-,32,8> 0.0, fxp<+/-,32,8> 0.0, fxp<+/-,32,8> 0.0, fxp<+/-,32,8> 0.0) -> (w258:fxp<+/-,32,8>[])
            "Mod5.Monitor" <- w258
            n106 = call "Analog_Output_16Channels_W20I5.vi"("Values"=w258, "IO"=T38 {"AO 0"="Mod5/AO0", "AO 1"="Mod5/AO1", "AO 2"="Mod5/AO2", "AO 3"="Mod5/AO3", "AO 4"="Mod5/AO4", "AO 5"="Mod5/AO5", "AO 6"="Mod5/AO6", "AO 7"="Mod5/AO7", "AO 8"="Mod5/AO8", "AO 9"="Mod5/AO9", "AO 10"="Mod5/AO10", "AO 11"="Mod5/AO11", "AO 12"="Mod5/AO12", "AO 13"="Mod5/AO13", "AO 14"="Mod5/AO14", "AO 15"="Mod5/AO15"}) -> ()  [unwired: 1 in]
            "Actual Analog Output Loop Period (usec)" <- w333
          }
        }
      }
      n107 = node-c288() -> (w100:T32)  [unwired: 1 in]
      n108 = timed-loop "EST APU Loop" {
        timing: w98 -> [_]
        timing-out: [_] -> w97
        tunnel: w96 -> [w101]
        stop <- _ stop-if-true
        n109 = call "Angle Processing Unit.vi"("settings.<user name>"="settings.apu 1", "register bus"=w101, "input.<user name>"="input.apu 1") -> ("output.<user name>"=→"output.apu 1":T27)  [unwired: 8 in]
      }
      n110 = timed-loop "Digital High Speed Loop" {
        timing: w100 -> [_]
        timing-out: [_] -> w99
        tunnel: w96 -> [w113]
        tunnel: w93 -> [w112]
        tunnel: w92 -> [w111]
        tunnel: w91 -> [w110]
        tunnel: w90 -> [w109]
        stop <- _ stop-if-true
        n111 = flat-sequence "Timing Control" {
          tunnel: w113 -> [w198]
          tunnel: w112 -> [w199]
          tunnel: w111 -> [w195]
          tunnel: w110 -> [w192]
          tunnel: w109 -> [w189]
          frame #0 {
            n112 = call "Directional Speed Sensor.vi"("load data"=w189, "settings.<user name>"="settings.Crank", "register bus"=w198, "input.<user name>"="input.Crank") -> ("digial output"=w181:bool)  [unwired: 7 in]
            n113 = call "WSS.Generate.Digital.vi"("Settings"="Front Driver WS.Settings") -> ("Bit1"=w176:bool, "Bit0"=w177:bool)  [unwired: 8 in, 1 out]
            n114 = call "Digital_Input_8Channels.vi"("IO"=T35 {"DI 0"="Mod4/DIO0", "DI 1"="Mod4/DIO1", "DI 2"="Mod4/DIO2", "DI 3"="Mod4/DIO3", "DI 4"="Mod4/DIO4", "DI 5"="Mod4/DIO5", "DI 6"="Mod4/DIO6", "DI 7"="Mod4/DIO7"}) -> ("States"=w123:bool[])
            "Mod4.Monitor" <- w123
            n115 = call "PWM.Generate.Digital.vi"("Settings"="PWM Out 1.Settings") -> ("Output"=w188:bool)  [unwired: 10 in]
            n116 = call "PWM.Generate.Digital.vi"("Settings"="PWM Out 2.Settings") -> ("Output"=w187:bool)  [unwired: 10 in]
            n117 = call "Digital Pattern Generation.vi"("load data"=w199, "settings.<user name>"="settings.Intake CAM 1", "register bus"=w198, "input.<user name>"="input.Intake CAM 1") -> ("digial output"=w186:bool)  [unwired: 7 in]
            n118 = call "Digital Pattern Generation.vi"("load data"=w195, "settings.<user name>"="settings.Exhaust CAM 1", "register bus"=w198, "input.<user name>"="input.Exhaust CAM 1") -> ("digial output"=w185:bool)  [unwired: 7 in]
            n119 = call "Digital Pattern Generation.vi"("load data"=w192, "settings.<user name>"="settings.Crank_Temp", "register bus"=w198, "input.<user name>"="input.Crank_Temp") -> ("digial output"=w182:bool)  [unwired: 7 in]
            n120 = call "Digital_Input_8Channels.vi"("IO"=T35 {"DI 0"="Mod3/DIO0", "DI 1"="Mod3/DIO1", "DI 2"="Mod3/DIO2", "DI 3"="Mod3/DIO3", "DI 4"="Mod3/DIO4", "DI 5"="Mod3/DIO5", "DI 6"="Mod3/DIO6", "DI 7"="Mod3/DIO7"}) -> ("States"=w163:bool[])
            "Mod3.Monitor" <- w163
            n121 = call "Static.Generate.Digital.vi"("Settings"="Accessory.Settings") -> ("Output"=w172:bool)  [unwired: 10 in]
            n122 = call "Static.Generate.Digital.vi"("Settings"="Ign Power.Settings") -> ("Output"=w171:bool)  [unwired: 10 in]
            n123 = Build Array(w177, w176) -> (w173:bool[])
            n124 = Index Array(array=w123) -> (element #1=w121:bool, element #3=w118:bool, element #4=w115:bool)  [unwired: 8 in, 5 out]
            n125 = Index Array(array=w163) -> (element #1=w161:bool, element #2=w158:bool, element #3=w155:bool, element #4=w143:bool, element #5=→"Key Loopback":bool, element #6=→"Switch Loopback":bool, element #7=w129:bool, element #8=w126:bool)  [unwired: 8 in]
            n126 = Build Array(w188, w187, w186, w185, "Key", "Switch", w182, w181) -> (w179:bool[])
            "Mod1.Monitor" <- w179
            n127 = call "Static.Measure.Digital.vi"("State"=w121, "Settings"="Front Driver WS Loopback.Settings") -> ("Measurement"=→"Front Driver WS Loopback.Measure":T1)  [unwired: 9 in]
            n128 = call "Static.Measure.Digital.vi"("State"=w115, "Settings"="Ign Power Loopback.Settings") -> ("Measurement"=→"Ign Power Loopback.Measure":T1)  [unwired: 9 in]
            n129 = call "Static.Measure.Digital.vi"("State"=w118, "Settings"="Accessory Loopback.Settings") -> ("Measurement"=→"Accessory Loopback.Measure":T1)  [unwired: 9 in]
            n130 = call "PWM.Measure.Digital.vi"("State"=w158, "Settings"="PWM Out 2 Loopback.Settings") -> ("Measurement"=→"PWM Out 2 Loopback.Measure":T6)  [unwired: 8 in, 1 out]
            n131 = call "PWM.Measure.Digital.vi"("State"=w161, "Settings"="PWM Out 1 Loopback.Settings") -> ("Measurement"=→"PWM Out 1 Loopback.Measure":T6)  [unwired: 8 in, 1 out]
            n132 = call "Static.Measure.Digital.vi"("State"=w129, "Settings"="Crank_Temp Loopback.Settings") -> ("Measurement"=→"Crank_Temp Loopback.Measure":T1)  [unwired: 9 in]
            n133 = call "Static.Measure.Digital.vi"("State"=w126, "Settings"="Crank Loopback.Settings") -> ("Measurement"=→"Crank Loopback.Measure":T1)  [unwired: 9 in]
            n134 = call-poly "Measure Events.vi"("settings.<user name>"="settings.Exhaust CAM 1 Loopback", "register bus"=w198, "event"=w143) -> ("measured data"=w140:T44, "status.<user name>"=→"status.Exhaust CAM 1 Loopback":T4)  [unwired: 7 in]
            n135 = call-poly "Measure Events.vi"("settings.<user name>"="settings.Intake CAM 1 Loopback", "register bus"=w198, "event"=w155) -> ("measured data"=w152:T44, "status.<user name>"=→"status.Intake CAM 1 Loopback":T4)  [unwired: 7 in]
            n136 = Build Array (concatenate)(w173, w172, w171, FALSE, FALSE, FALSE, FALSE) -> (w165:bool[])
            "Mod2.Monitor" <- w165
            n137 = call "Digital_Output_8Channels.vi"("States"=w179, "IO"=T37 {"DO 0"="Mod1/DIO0", "DO 1"="Mod1/DIO1", "DO 2"="Mod1/DIO2", "DO 3"="Mod1/DIO3", "DO 4"="Mod1/DIO4", "DO 5"="Mod1/DIO5", "DO 6"="Mod1/DIO6", "DO 7"="Mod1/DIO7"}) -> ()  [unwired: 1 in]
            n138 = call "Capture Event.vi"("event # to capture"=T36 1, "measured data"=w140) -> ("capture.<user name>"=→"capture.Exhaust CAM 1 Loopback.Event 1":T3)  [unwired: 9 in]
            n139 = call "Capture Event.vi"("event # to capture"=T36 2, "measured data"=w140) -> ("capture.<user name>"=→"capture.Exhaust CAM 1 Loopback.Event 2":T3)  [unwired: 9 in]
            n140 = call "Capture Event.vi"("event # to capture"=T36 3, "measured data"=w140) -> ("capture.<user name>"=→"capture.Exhaust CAM 1 Loopback.Event 3":T3)  [unwired: 9 in]
            n141 = call "Capture Event.vi"("event # to capture"=T36 4, "measured data"=w140) -> ("capture.<user name>"=→"capture.Exhaust CAM 1 Loopback.Event 4":T3)  [unwired: 9 in]
            n142 = call "Capture Event.vi"("event # to capture"=T36 1, "measured data"=w152) -> ("capture.<user name>"=→"capture.Intake CAM 1 Loopback.Event 1":T3)  [unwired: 9 in]
            n143 = call "Capture Event.vi"("event # to capture"=T36 2, "measured data"=w152) -> ("capture.<user name>"=→"capture.Intake CAM 1 Loopback.Event 2":T3)  [unwired: 9 in]
            n144 = call "Capture Event.vi"("event # to capture"=T36 3, "measured data"=w152) -> ("capture.<user name>"=→"capture.Intake CAM 1 Loopback.Event 3":T3)  [unwired: 9 in]
            n145 = call "Capture Event.vi"("event # to capture"=T36 4, "measured data"=w152) -> ("capture.<user name>"=→"capture.Intake CAM 1 Loopback.Event 4":T3)  [unwired: 9 in]
            n146 = call "Digital_Output_8Channels.vi"("States"=w165, "IO"=T37 {"DO 0"="Mod2/DIO0", "DO 1"="Mod2/DIO1", "DO 2"="Mod2/DIO2", "DO 3"="Mod2/DIO3", "DO 4"="Mod2/DIO4", "DO 5"="Mod2/DIO5", "DO 6"="Mod2/DIO6", "DO 7"="Mod2/DIO7"}) -> ()  [unwired: 1 in]
          }
        }
      }
      n147 = node-c288 ("Output Node")(w97) -> ()
      n148 = node-c288 ("Output Node")(w99) -> ()
    }
  }
